vi "Queue_GEA2_Brass.vi"(0 "Output String":string, 11 "error in (no error)":errorcluster) -> (15 "error out":errorcluster)   [LabVIEW 2016]
uses:
  Common/GExplorer Support/typedefs/GExplorer_Data_Cluster.ctl
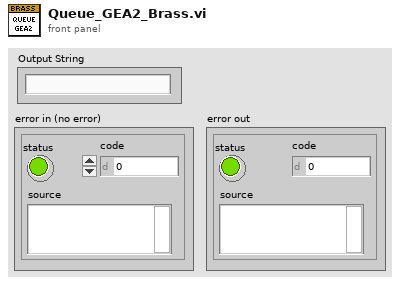
[diagram p1: front panel]
types:
  T1 = typedef "GExplorer_Data_Cluster.ctl" = cluster{"Data":variant, "State":enum16{"Add to Log", "Clear", "Shutdown"}}
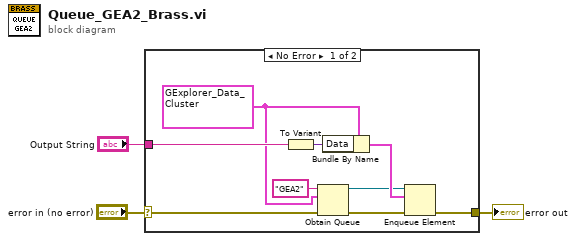
[diagram p0: block diagram]
diagram:
  n1 = case shown="No Error" "error in (no error)" {
    selector: "error in (no error)" -> [w9 w13]
    tunnel: [w4 w13] -> w3
    tunnel: "Output String" -> [w10 _]
    frame No Error {
      w5 = T1 {"Data"=variant, "State"=enum."Add to Log"} ("Data")
      n2 = To Variant(anything=w10) -> (Variant=w11:variant)
      n3 = Obtain Queue(name (unnamed)="GEA2", element data type=w5, error in (no error)=w9) -> (queue out=w7:refnum<queue>, error out=w8:errorcluster)  [unwired: 2 in, 1 out]
      n4 = Bundle By Name(cluster=w5, "Data"=w11) -> (w12:T1)
      n5 = Enqueue Element(queue=w7, element=w12, error in (no error)=w8) -> (error out=w4:errorcluster)  [unwired: 1 in, 2 out]
    }
    frame Error {
    }
  }
  "error out" <- w3
